vi "background process.vi"(11 "communication refs":T1) -> ()   [LabVIEW 2013, in "worker pool.lvlib"]
uses:
  worker pool.lvlib
  worker comms.ctl
  worker commands.ctl
  request fifos.ctl
  recovery request.ctl
  <vilib>/NI/Tag Bus Module Framework/runtime/TBM module execution interface.lvclass
  <vilib>/NI/Tag Bus Module Framework/module configuration/TBM module configuration.lvclass
  response fifos.ctl
  recovery response.ctl
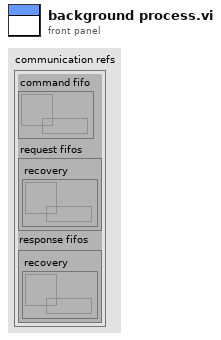
[diagram p1: front panel]
types:
  T1 = typedef "worker pool.lvlib/worker comms.ctl" = cluster{"command fifo":refnum<k33>, "request fifos":T2, "response fifos":T3}
  T2 = typedef "worker pool.lvlib/request fifos.ctl" = cluster{"recovery":refnum<k33>}
  T3 = typedef "worker pool.lvlib/response fifos.ctl" = cluster{"recovery":refnum<k33>}
  T4 = typedef "worker pool.lvlib/worker commands.ctl" = enum16{"shutdown", "recover module"}
  T5 = typedef "worker pool.lvlib/recovery request.ctl" = cluster{"module ref":refnum<data-value>, "engine reference":i32, "original run flags":u8, "attempts allowed":u16, "cfg ref":refnum<data-value>}
  T6 = typedef "worker pool.lvlib/recovery response.ctl" = cluster{"module ref":refnum<data-value>, "engine reference":i32, "original run flags":u8, "success?":bool, "error code":i32}
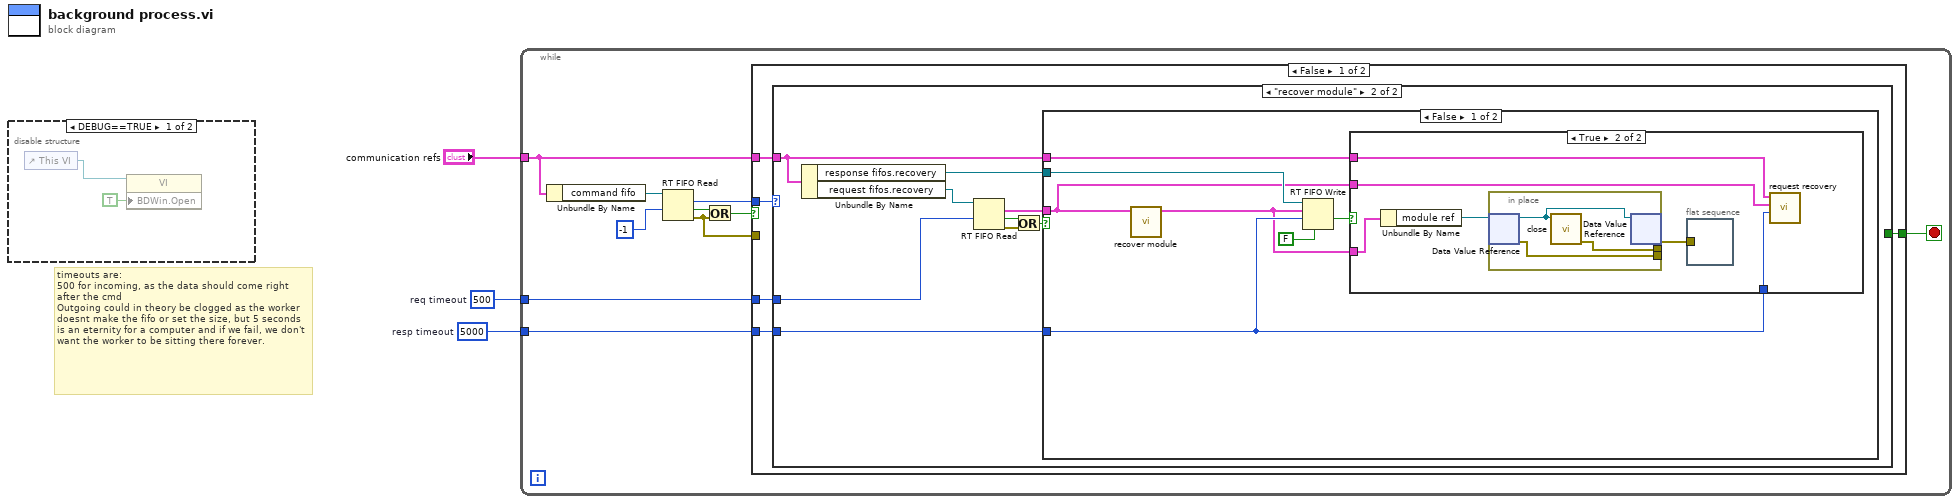
[diagram p0: block diagram]
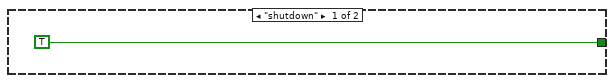
[diagram p3: hidden frame]
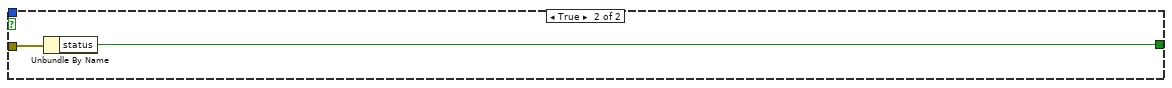
[diagram p6: hidden frame]
diagram:
  w1 = 5000  # resp timeout
  w2 = 500  # req timeout
  # "timeouts are:\n500 for incoming, as the data should come right after the cmd\nOutgoing could in theory be clogged as the worker doesnt make the fifo or set the size, but 5 seconds is an eternity for a computer and if we fail, we don't want the worker to be sitting there forever."
  n1 = disable-structure shown="DEBUG==TRUE" {
    frame condition #0 {
      n2 = control-ref of="This VI"() -> (w5:refnum<vi>)
      n3 = property class="VI"(reference=w5, "BDWin.Open"=TRUE ("Block Diagram Window:Open")) -> ()  [unwired: 1 in, 2 out]
    }
    frame condition #1 (active) {
    }
  }
  n4 = while {
    tunnel: "communication refs" -> [w8]
    tunnel: w2 -> [w7]
    tunnel: w1 -> [w6]
    stop <- w11 stop-if-true
    n5 = Unbundle By Name(w8) -> ("command fifo"=w15:refnum<k33>)
    n6 = RT FIFO Read(0:w15, 2:-1 ("timeout in ms (0)")) -> (9:w9:T4, 10:w14:bool, 11:w12:errorcluster)  [unwired: 2 in, 2 out]
    n7 = Or(x=w14, y=w12) -> (x .or. y?=w13:bool)
    n8 = case shown="False" w13 {
      tunnel: w12 -> [_ w48]
      tunnel: [w19 w47] -> w11
      tunnel: w9 -> [w20 _]
      tunnel: w8 -> [w18 _]
      tunnel: w7 -> [w17 _]
      tunnel: w6 -> [w16 _]
      frame False {
        n9 = case shown="\"recover module\"" w20 {
          tunnel: [TRUE _] -> w19
          tunnel: w18 -> [_ w22]
          tunnel: w17 -> [_ w24]
          tunnel: w16 -> [_ w23]
          frame "shutdown" {
          }
          frame "recover module" {
            n10 = Unbundle By Name(w22) -> ("response fifos.recovery"=w25:refnum<k33>, "request fifos.recovery"=w30:refnum<k33>)
            n11 = RT FIFO Read(0:w30, 2:w24) -> (9:w26:T5, 10:w29:bool, 11:w28:errorcluster)  [unwired: 2 in, 2 out]
            n12 = Or(x=w29, y=w28) -> (x .or. y?=w27:bool)
            n13 = case shown="False" w27 {
              tunnel: w26 -> [w32 _]
              tunnel: w25 -> [w37 _]
              tunnel: w23 -> [w33 _]
              tunnel: w22 -> [w34 _]
              frame False {
                n14 = call "recover module.vi"("recovery request"=w32) -> ("response"=w31:T6)  [unwired: 10 in]
                n15 = RT FIFO Write(0:w37, 1:w31, 2:w33, 5:FALSE ("overwrite on timeout (T)")) -> (10:w35:bool)  [unwired: 1 in, 3 out]
                n16 = case shown="True" w35 {
                  tunnel: w34 -> [_ w43]
                  tunnel: w33 -> [_ w42]
                  tunnel: w32 -> [_ w41]
                  tunnel: w31 -> [_ w40]
                  frame False {
                  }
                  frame True {
                    n17 = Unbundle By Name(w40) -> ("module ref"=w39:refnum<data-value>)
                    n18 = in-place {
                      in-place-border: [w45] -> _
                      in-place-border: [w44] -> _
                      n19 = in-place-dvr #1(w39) -> (w46:refnum<class "TBM module execution interface.lvclass">, w44:errorcluster)
                      n20 = call-dynamic "close.vi"("module in"=w46) -> ("error out"=w45:errorcluster)  [unwired: 10 in]
                      n21 = in-place-dvr #1(w46) -> (w38:errorcluster)  [unwired: 1 out]
                    }
                    n22 = flat-sequence {
                      tunnel: w38 -> [_]
                      frame #0 {
                      }
                    }
                    n23 = call "request recovery.vi"("timeout in ms (0)"=w42, "recovery request"=w41, "worker comms in"=w43) -> ()  [unwired: 8 in, 1 out]
                  }
                }
              }
              frame True {
              }
            }
          }
        }
      }
      frame True {
        n24 = Unbundle By Name(w48) -> ("status"=w47:bool)
      }
    }
  }
